vi "Get Calibration.vi"(8 "error in (no error)":errorcluster, 11 "DAQmx in":refnum<class "DAQmx.lvclass">) -> (0 "error out":errorcluster, 2 "Calibration":T1 {"DevTemp" format="%.1f"; "SelfCal.LastTemp" format="%.1f"; "SelfCal.LastDate/Time" format="%<%I:%M %p %m/%d/%Y>T"}, 3 "DAQmx out":refnum<class "DAQmx.lvclass">)   [LabVIEW 2019, in "DAQmx.lvclass"]
uses:
  DAQmx.lvclass
  typedefs/DAQ.Calibration--Cluster--Array.ctl
  typedefs/DAQ.Calibration--Cluster.ctl
  DAQmx.lvclass/DAQmx.ctl
  <resource>/objmgr/daqmx.rc
panel:
  out "cal due?":bool
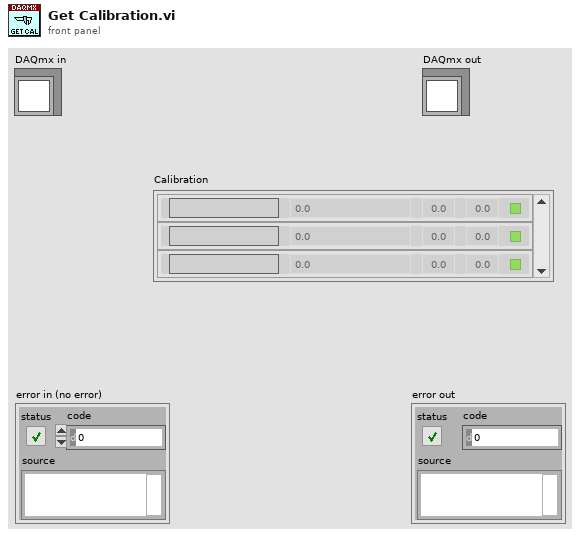
[diagram p1: front panel]
types:
  T1 = typedef "DAQmx.lvclass/DAQ.Calibration--Cluster--Array.ctl" = T2[]
  T2 = typedef "DAQmx.lvclass/DAQ.Calibration--Cluster.ctl" = cluster{"Active Device":string, "SelfCal.LastDate/Time":dbl, "SelfCal.LastTemp":dbl, "DevTemp":dbl, "calibration due?":bool}
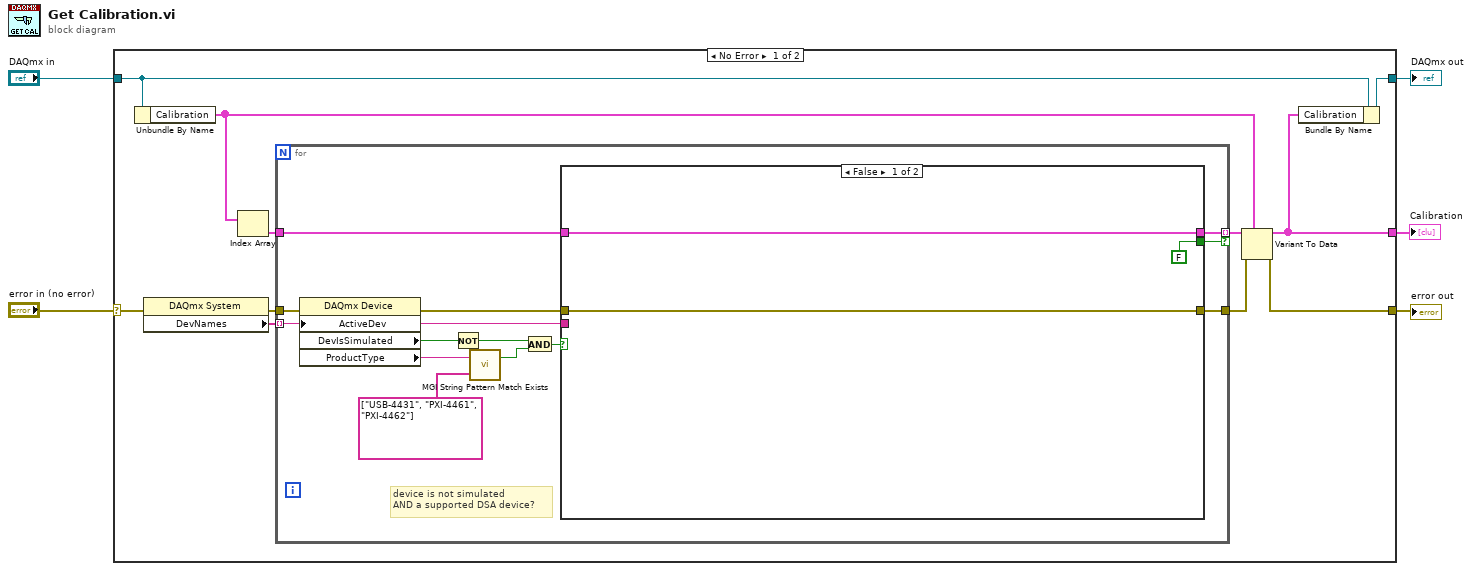
[diagram p0: block diagram]
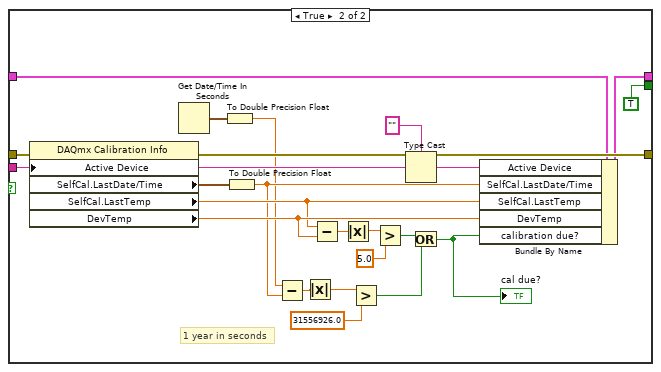
[diagram p2: hidden frame]
diagram:
  n1 = case shown="No Error" "error in (no error)" {
    selector: "error in (no error)" -> [w13 w56]
    tunnel: [w7 w56] -> w5
    tunnel: "DAQmx in" -> [w12 w57]
    tunnel: [w16 w57] -> w3
    tunnel: [w8 _] -> w2
    frame No Error {
      n2 = Unbundle By Name(w12) -> ("Calibration"=w10:T1)
      n3 = property class="DAQmx System"(error in=w13) -> (error out=w14:errorcluster, "DevNames"=w15:tag[])  [unwired: 1 in, 1 out]
      n4 = Index Array(array=w10) -> (element=w11:T2)  [unwired: 1 in]
      n5 = for {
        tunnel: [w28] -> w9 mode=indexing if=w19
        tunnel: w15 -> [w26] mode=indexing
        tunnel: w11 -> [w17]
        tunnel: w14 -> [w27]
        tunnel: [w29] -> w6
        # "device is not simulated\nAND a supported DSA device?"
        n6 = property class="DAQmx Device"(error in=w27, "ActiveDev"=w26) -> (error out=w25:errorcluster, "DevIsSimulated"=w24:bool, "ProductType"=w21:string)  [unwired: 1 in, 1 out]
        n7 = Not(x=w24) -> (.not. x?=w22:bool)
        n8 = call <userlib>:"MGI String Pattern Match Exists.vi"("Patterns to Try"=string[] ["USB-4431", "PXI-4461", "PXI-4462"], "String"=w21) -> ("Match Found"=w20:bool)  [unwired: 1 out]
        n9 = And(x=w22, y=w20) -> (x .and. y?=w23:bool)
        n10 = case shown="False" w23 {
          tunnel: [w32 w55] -> w29
          tunnel: [w30 w41] -> w28
          tunnel: w26 -> [_ w43]
          tunnel: w25 -> [w32 w42]
          tunnel: [FALSE TRUE] -> w19
          tunnel: w17 -> [w30 w40]
          frame False {
          }
          frame True {
            # "1 year in seconds"
            n11 = property class="DAQmx Calibration Info"(error in=w42, "Active Device"=w43) -> (error out=w55:errorcluster, "SelfCal.LastDate/Time"=w49:timestamp, "SelfCal.LastTemp"=w50:dbl, "DevTemp"=w51:dbl)  [unwired: 1 in, 1 out]
            n12 = Get Date/Time In Seconds() -> (seconds since 1Jan1904=w37:timestamp)
            n13 = To Double Precision Float(number=w37) -> (double precision float=w35:dbl)
            n14 = To Double Precision Float(number=w49) -> (double precision float=w36:dbl)
            n15 = Subtract(x=w35, y=w36) -> (x-y=w48:dbl)
            n16 = Absolute Value(x=w48) -> (abs(x)=w47:dbl)
            n17 = Subtract(x=w50, y=w51) -> (x-y=w54:dbl)
            n18 = Absolute Value(x=w54) -> (abs(x)=w53:dbl)
            n19 = Greater?(x=w47, y=31556926.0) -> (0:w45:bool)
            n20 = Greater?(x=w53, y=5.0) -> (0:w46:bool)
            n21 = Type Cast(type="", x=w43) -> (*(type *) &x=w34:string)
            n22 = Or(x=w46, y=w45) -> (x .or. y?=w38:bool)
            "cal due?" <- w38
            n23 = Bundle By Name(cluster=w40, "Active Device"=w34, "SelfCal.LastDate/Time"=w36, "SelfCal.LastTemp"=w50, "DevTemp"=w51, "calibration due?"=w38) -> (w41:T2)
          }
        }
      }
      n24 = Variant To Data(error in=w6, type=w10, Variant=w9) -> (data=w8:T1, error out=w7:errorcluster)
      n25 = Bundle By Name(cluster=w12, "Calibration"=w8) -> (w16:refnum<class "DAQmx.lvclass">)
    }
    frame Error {
    }
  }
  "error out" <- w5
  "Calibration" <- w2
  "DAQmx out" <- w3
